vi "get duty cycle.vi"(8 "error in (no error)":errorcluster, 11 "ImagingModeSPIM in":refnum<class "ImagingModeSPIM.lvclass">) -> (0 "error out":errorcluster, 3 "ImagingModeSPIM out":refnum<class "ImagingModeSPIM.lvclass">)   [LabVIEW 2012, in "ImagingModeSPIM.lvclass"]
uses:
  ImagingModeSPIM.lvclass
  ImagingModeSPIM.lvclass/ImagingModeSPIM.ctl
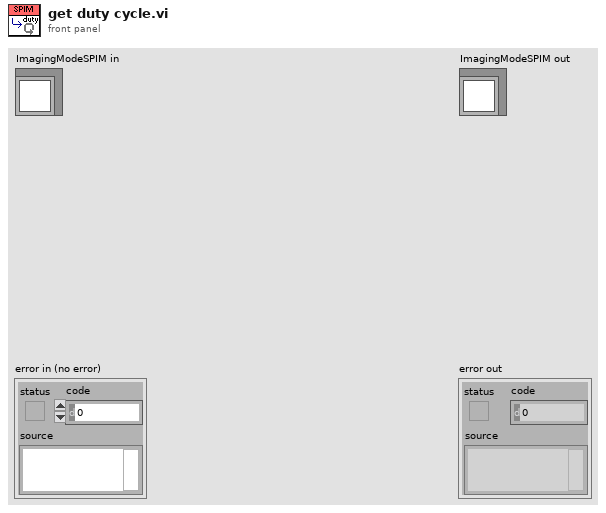
[diagram p1: front panel]
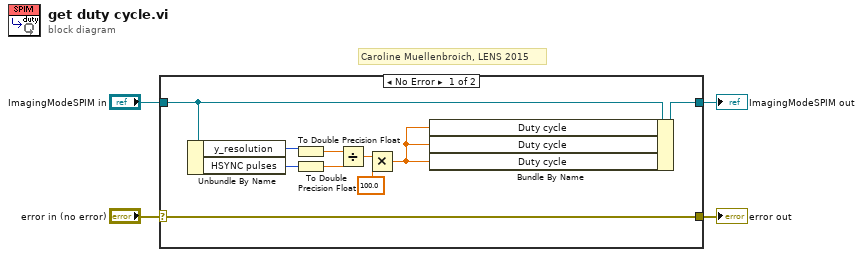
[diagram p0: block diagram]
diagram:
  # "Caroline Muellenbroich, LENS 2015"
  n1 = case shown="No Error" "error in (no error)" {
    selector: "error in (no error)" -> [w14 w16]
    tunnel: [w14 w16] -> w3
    tunnel: [w7 w15] -> w1
    tunnel: "ImagingModeSPIM in" -> [w8 w15]
    frame No Error {
      n2 = Unbundle By Name(w8) -> ("y_resolution"=w10:i32, "HSYNC pulses"=w6:i32)
      n3 = To Double Precision Float(number=w10) -> (double precision float=w11:dbl)
      n4 = To Double Precision Float(number=w6) -> (double precision float=w5:dbl)
      n5 = Divide(x=w11, y=w5) -> (x/y=w12:dbl)
      n6 = Multiply(x=w12, y=100.0) -> (x*y=w9:dbl)
      n7 = Bundle By Name(cluster=w8, "Duty cycle"=w9, "Duty cycle"=w9, "Duty cycle"=w9) -> (w7:refnum<class "ImagingModeSPIM.lvclass">)
    }
    frame Error {
    }
  }
  "error out" <- w3
  "ImagingModeSPIM out" <- w1
